vi "SOAE-Load Data.vi"(0 "selected path":path, 11 "error in (no error)":errorcluster) -> (4 "selected path out":path, 6 "Params":T1, 8 "data":cluster{dbl[], dbl[]}, 15 "error out":errorcluster)   [LabVIEW 2020]
uses:
  Typedefs/SOAE-Parameters.ctl
  <vilib>/regexp/Match Regular Expression.xnode
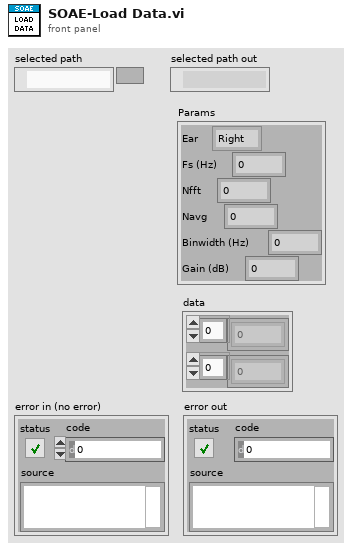
[diagram p1: front panel]
types:
  T1 = typedef "SOAE-Parameters.ctl" = cluster{"Ear":enum16{"Right", "Left"}, "Fs (Hz)":dbl, "Nfft":i32, "Navg":i32, "Binwidth (Hz)":dbl, "Gain (dB)":dbl}
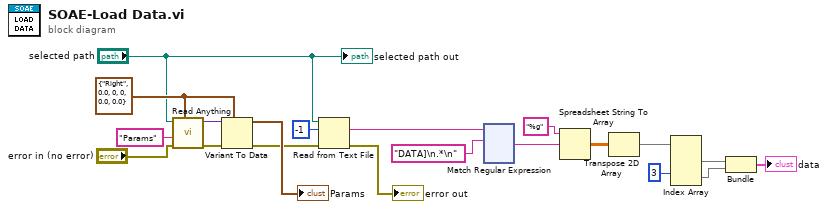
[diagram p0: block diagram]
diagram:
  w13 = T1 {"Ear"=enum."Right", "Fs (Hz)"=0.0, "Nfft"=0, "Navg"=0, "Binwidth (Hz)"=0.0, "Gain (dB)"=0.0} ("Params")
  n1 = call "Read Anything.vi"("Type of Anything"=w13, "Error In"="error in (no error)", "Section Name (Name of \"Type of Anything\")"="Params" ("Section Name (Name of \"Type of Anything\")"), "Path (dialog)"="selected path") -> ("Error Out"=w19:errorcluster, "Anything"=w20:variant)  [unwired: 5 in, 1 out]
  n2 = Variant To Data(error in=w19, type=w13, Variant=w20) -> (data=→"Params":T1, error out=w11:errorcluster)
  n3 = Read from Text File(file (use dialog)="selected path", count=-1, error in=w11) -> (text=w8:string, error out=→"error out":errorcluster)  [unwired: 1 in, 2 out]
  n4 = xnode "Match Regular Expression"("input string"=w8, "regular expression"="DATA]\n.*\n" ("search string/char (-)")) -> ("after match"=w1:string)  [unwired: 4 in, 4 out]
  n5 = Spreadsheet String To Array(format string="%g", spreadsheet string=w1) -> (array=w18:dbl[][])  [unwired: 2 in]
  n6 = Transpose 2D Array(2D array=w18) -> (transposed array=w6:dbl[][])
  n7 = Index Array(array=w6, index (row) #2=3 ("disabled index (col)")) -> (element #1=w5:dbl[], element #2=w3:dbl[])  [unwired: 3 in]
  n8 = Bundle(w5, w3) -> (→"data":cluster{dbl[], dbl[]})  [unwired: 1 in]
  "selected path out" <- "selected path"
